vi "Set Offset.vi"(8 "error in (no error)":errorcluster, 9 "set offset (F:no)":bool, 11 "VISA resource name":refnum<visa-resource-name>) -> (0 "error out":errorcluster, 3 "VISA resource name out":refnum<visa-resource-name>)   [LabVIEW 2009, in "Fluke 8840.lvlib"]
doc: "This VI allows the user to set/cancel the present reading as an offset for the present function."
uses:
  Fluke 8840.lvlib
panel:
  # "yes\nno"
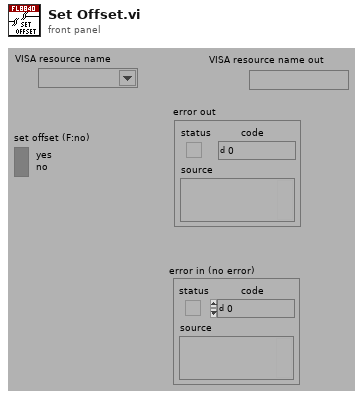
[diagram p1: front panel]
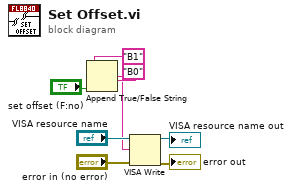
[diagram p0: block diagram]
diagram:
  n1 = Append True/False String(1:"set offset (F:no)", 2:"B0", 3:"B1") -> (0:w1:string)  [unwired: 1 out]
  n2 = VISA Write(VISA resource name="VISA resource name", write buffer=w1, error in (no error)="error in (no error)") -> (VISA resource name out=→"VISA resource name out":refnum<visa-resource-name>, error out=→"error out":errorcluster)  [unwired: 1 out]
